vi "CliCommandReceived.vi"(8 "error in (no error)":errorcluster, 10 "CommandReceived":refnum<class "CommandReceived.lvclass">, 11 "CallerMessage in":refnum<class "CallerMessage.lvclass">) -> (0 "error out":errorcluster, 3 "CallerMessage out":refnum<class "CallerMessage.lvclass">)   [LabVIEW 2022 SP3, in "Cli.lvlib" / "CallerMessage.lvclass"]
uses:
  CallerMessage.lvclass
  CommandReceived/CommandReceived.lvclass
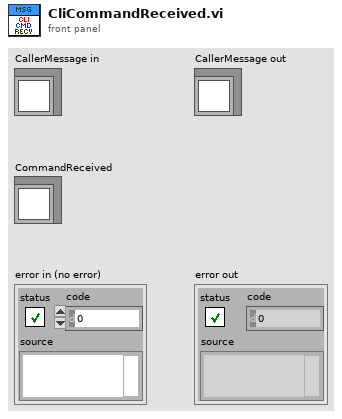
[diagram p1: front panel]
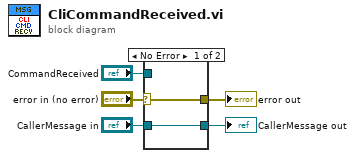
[diagram p0: block diagram]
diagram:
  n1 = case shown="No Error" "error in (no error)" {
    selector: "error in (no error)" -> [w6 w9]
    tunnel: [w6 w9] -> w4
    tunnel: [w7 w8] -> w2
    tunnel: "CallerMessage in" -> [w7 w8]
    tunnel: "CommandReceived" -> [_ _]
    frame No Error {
    }
    frame Error {
    }
  }
  "error out" <- w4
  "CallerMessage out" <- w2
